vi "Read Autoshutdown.vi"(8 "error in (no error)":errorcluster, 11 "RQMHStartup in":refnum<class "ModuleStartup.lvclass">) -> (0 "error out":errorcluster, 2 "Autostop?":bool, 3 "RQMHStartup out":refnum<class "ModuleStartup.lvclass">)   [LabVIEW 2024, in "ModuleStartup.lvclass"]
uses:
  ModuleStartup.lvclass
  ModuleStartup.lvclass/ModuleStartup.ctl
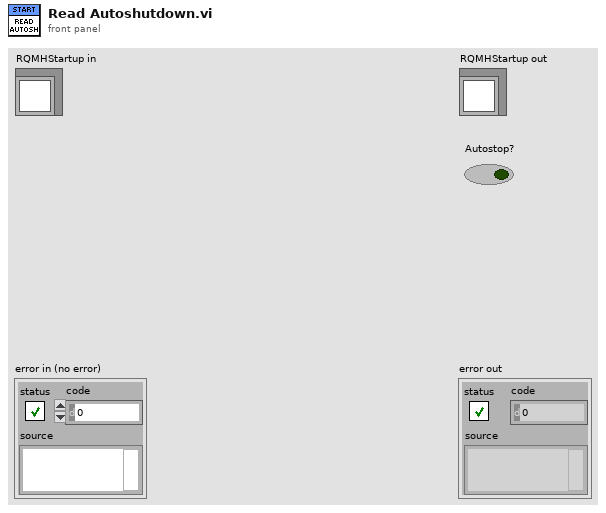
[diagram p1: front panel]
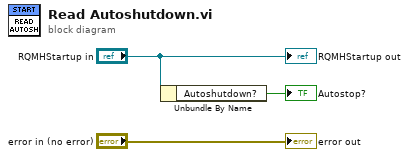
[diagram p0: block diagram]
diagram:
  n1 = Unbundle By Name("RQMHStartup in") -> ("Autoshutdown?"=→"Autostop?":bool)
  "error out" <- "error in (no error)"
  "RQMHStartup out" <- "RQMHStartup in"
